vi "Function.vi"(8 "error in (no error)":errorcluster, 9 "Numeric B":sgl, 10 "Numeric A":sgl, 11 "Two Terminal in":refnum<class "Not Equal_SGL.lvclass">) -> (0 "error out":errorcluster, 2 "Result":bool, 3 "Two Terminal out":refnum<class "Not Equal_SGL.lvclass">)   [LabVIEW 2021, in "Not Equal_SGL.lvclass"]
uses:
  Not Equal_SGL.lvclass
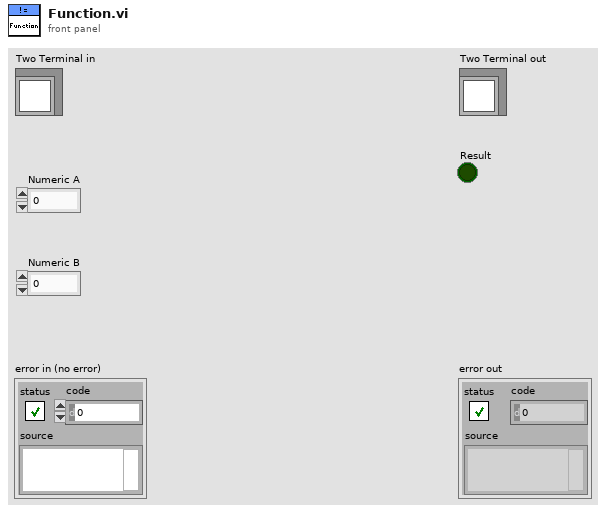
[diagram p1: front panel]
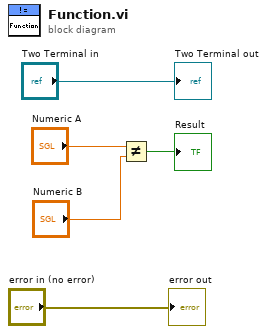
[diagram p0: block diagram]
diagram:
  n1 = Not Equal?(x="Numeric A", y="Numeric B") -> (x != y?=→"Result":bool)
  "error out" <- "error in (no error)"
  "Two Terminal out" <- "Two Terminal in"
